vi "ASCII to HEX.vi"(1 "String in ASCII":string) -> (0 "String in HEX":string)   [LabVIEW 2017]
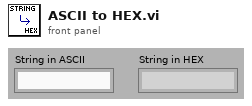
[diagram p1: front panel]
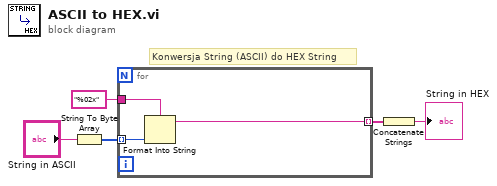
[diagram p0: block diagram]
diagram:
  # "Konwersja String (ASCII) do HEX String"
  n1 = String To Byte Array(string="String in ASCII") -> (unsigned byte array=w1:u8[])
  n2 = for {
    tunnel: w1 -> [w8] mode=indexing
    tunnel: "%02x" ("format string") -> [w7]
    tunnel: [w6] -> w3 mode=indexing
    n3 = Format Into String(format string=w7, w8) -> (resulting string=w6:string)  [unwired: 2 in, 1 out]
  }
  n4 = Concatenate Strings(w3) -> (→"String in HEX":string)
